vi "LEDTesting.vi"() -> ()   [LabVIEW 2014]
uses:
  <vilib>/myRIO/Instrument Drivers/Onboard IO/DIO/typedefs/DIO Reference.ctl
  <vilib>/myRIO/Common/Instrument Driver Framework/Utilities/typedefs/myRIO Generic Hardware Reference.ctl
  <vilib>/myRIO/Common/Instrument Driver Framework/Utilities/typedefs/Hardware Version Enum.ctl
  <vilib>/myRIO/Common/Instrument Driver Framework/Utilities/typedefs/myRIO v1.0 Reference.ctl
  <vilib>/myRIO/Common/Instrument Driver Framework/Utilities/typedefs/Generic FPGA Reference.ctl
  <vilib>/myRIO/Common/Instrument Driver Framework/myRIO v1.0/DIO/typedefs/DIO Channels List.ctl
  <vilib>/myRIO/Common/Instrument Driver Framework/myRIO v1.0/DIO/typedefs/DIO Channels Enum.ctl
  <vilib>/userdefined/High Color/nirio_resource_hc.ctl
  <vilib>/myRIO/Common/Instrument Driver Framework/Utilities/vis/Is FPGA Ref Available.vi
  <vilib>/myRIO/Common/Instrument Driver Framework/myRIO v1.0/DIO/vis/myRIO v1.1 Open DIO.vi
  <vilib>/myRIO/Instrument Drivers/Onboard IO/DIO/vis/Read.vi
  <vilib>/myRIO/Instrument Drivers/Onboard IO/DIO/vis/Write.vi
  <vilib>/myRIO/Common/Instrument Driver Framework/Utilities/vis/Validate Channels.vi
  <vilib>/myRIO/Common/Instrument Driver Framework/myRIO v1.0/DIO/vis/myRIO v1.0 Reserve DIO.vi
  <vilib>/myRIO/Common/Instrument Driver Framework/myRIO v1.0/Resource Manager/vis/myRIO v1.0 Reserve Channel List.vi
  <vilib>/myRIO/Common/Instrument Driver Framework/myRIO v1.0/DIO/vis/myRIO v1.0 Build MUX Configuration DIO.vi
  <vilib>/myRIO/Common/Instrument Driver Framework/myRIO v1.0/Resource Manager/vis/myRIO v1.0 Reserve Channel.vi
  <vilib>/myRIO/Common/Instrument Driver Framework/myRIO v1.0/Resource Manager/vis/myRIO v1.0 Unreserve Channel.vi
  <vilib>/myRIO/Common/Instrument Driver Framework/myRIO v1.0/Resource Manager/vis/myRIO v1.0 Create Configuration List.vi
  <vilib>/myRIO/Common/Instrument Driver Framework/myRIO v1.0/Resource Manager/vis/myRIO v1.0 Build Mutex Name.vi
  <vilib>/Utility/VariantDataType/GetNumericInfo.vi
  <vilib>/Utility/error.llb/Error Cluster From Error Code.vi
  <vilib>/myRIO/Common/Instrument Driver Framework/myRIO v1.0/myRIO v1.1 Open.vi
  <vilib>/myRIO/Common/Instrument Driver Framework/Utilities/vis/IO Manager.vi
  <vilib>/myRIO/Common/Instrument Driver Framework/Utilities/vis/Configuration Manager.vi
  <vilib>/myRIO/Common/Instrument Driver Framework/myRIO v1.0/Resource Manager/vis/myRIO v1.0 Configure IO.vi
  <vilib>/myRIO/Common/Instrument Driver Framework/myRIO v1.0/myRIO v1.0 Close.vi
  <vilib>/myRIO/Common/Instrument Driver Framework/myRIO v1.0/DIO/vis/myRIO v1.0 Read DIO.vi
  <vilib>/myRIO/Common/Instrument Driver Framework/myRIO v1.0/DIO/vis/myRIO v1.0 Write DIO.vi
  <vilib>/myRIO/Express VI/Onboard IO/DI/DI Express VI.xnode
  <vilib>/myRIO/Instrument Drivers/Onboard IO/DIO/vis/myRIO DIO Open.xnode
  <vilib>/myRIO/Express VI/Onboard IO/DO/DO Express VI.xnode
  <vilib>/myRIO/Instrument Drivers/Onboard IO/DIO/DIO.lvlib
  <vilib>/ptbypt/NI_PtbyPt.lvlib
panel:
  in  "stop":bool
  out "Outlet 1 Mode":enum16{"Off", "On", "Auto"}(ring)=enum."Auto"
  in  "x+1 2":i32
  in  "stop 2":bool
  out "x+1":i32
  in  "Enum":enum16{"Off", "On", "Auto"}(ring)
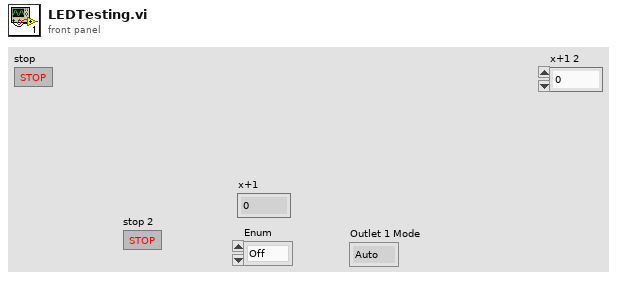
[diagram p1: front panel]
types:
  T1 = typedef "DIO.lvlib/DIO Reference.ctl" = cluster{"myRIO Reference":T2, "DIO Channels List":T6}
  T2 = typedef "myRIO Generic Hardware Reference.ctl" = cluster{"myRIO Model":T3, "myRIO Hardware Reference":T4}
  T3 = typedef "Hardware Version Enum.ctl" = enum16{"Unknown", "myRIO-1900", "myRIO-1950"}
  T4 = typedef "myRIO v1.0 Reference.ctl" = cluster{"Generic FPGA Reference":T5, "Allow multiple opens":bool}
  T5 = typedef "Generic FPGA Reference.ctl" = refnum<k20>
  T6 = typedef "DIO Channels List.ctl" = T7[]
  T7 = typedef "DIO Channels Enum.ctl" = enum16{"Not Connected", "C/DIO0", "C/DIO1", "C/DIO2", "C/DIO3", "C/DIO4", "C/DIO5", "C/DIO6", "C/DIO7", "A/DIO0", "A/DIO1", "A/DIO2", "A/DIO3", "A/DIO4", "A/DIO5", "A/DIO6", "A/DIO7", "A/DIO8", "A/DIO9", "A/DIO10", "A/DIO11", "A/DIO12", "A/DIO13", "A/DIO14", "A/DIO15", "B/DIO0", "B/DIO1", "B/DIO2", "B/DIO3", "B/DIO4", "B/DIO5", "B/DIO6", "B/DIO7", "B/DIO8", "B/DIO9", "B/DIO10", "B/DIO11", "B/DIO12", "B/DIO13", "B/DIO14", "B/DIO15", "LED0", "LED1", "LED2", "LED3", "Button0"}
  T8 = typedef "nirio_resource_hc.ctl" = tag
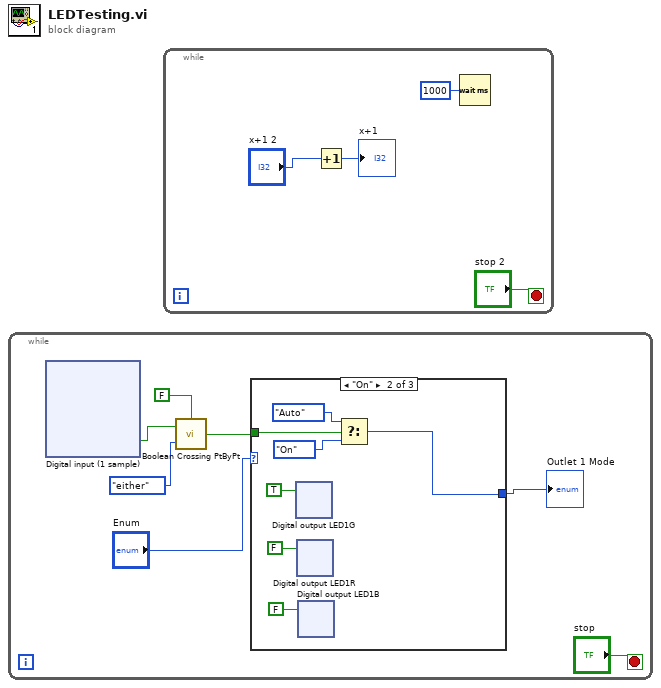
[diagram p0: block diagram]
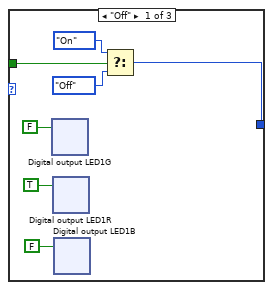
[diagram p2: hidden frame]
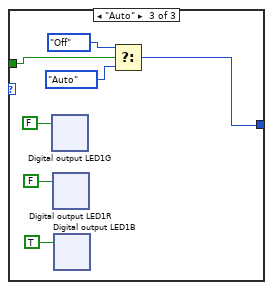
[diagram p3: hidden frame]
diagram:
  n1 = while {
    stop <- "stop" stop-if-true
    n2 = xnode "Digital input (1 sample)"() -> ("Button1 (B/DIO0 (Pin 11))"=w4:bool)  [unwired: 1 in, 1 out]
    n3 = call <vilib>:"Boolean Crossing PtByPt.vi"("initialize"=FALSE, "direction"=enum16{"either", "false-true", "true-false"}."either", "input"=w4) -> ("crossing"=w6:bool)
    n4 = case shown="\"On\"" "Enum" {
      tunnel: [w49 w161 w273] -> w3
      tunnel: w6 -> [w48 w158 w271]
      frame "Off" {
        n5 = xnode "Digital output LED1G"("LED1G (A/DIO0 (Pin 11))"=FALSE) -> ()  [unwired: 1 in, 1 out]
        n6 = xnode "Digital output LED1R"("LED1R (A/DIO1 (Pin 13))"=TRUE) -> ()  [unwired: 1 in, 1 out]
        n7 = xnode "Digital output LED1B"("LED1B (A/DIO2 (Pin 15))"=FALSE) -> ()  [unwired: 1 in, 1 out]
        n8 = Select(t=enum16{"Off", "On", "Auto"}."On", s=w48, f=enum16{"Off", "On", "Auto"}."Off") -> (s? t:f=w49:enum16{"Off", "On", "Auto"})
      }
      frame "On" {
        n9 = xnode "Digital output LED1G"("LED1G (A/DIO0 (Pin 11))"=TRUE) -> ()  [unwired: 1 in, 1 out]
        n10 = xnode "Digital output LED1R"("LED1R (A/DIO1 (Pin 13))"=FALSE) -> ()  [unwired: 1 in, 1 out]
        n11 = xnode "Digital output LED1B"("LED1B (A/DIO2 (Pin 15))"=FALSE) -> ()  [unwired: 1 in, 1 out]
        n12 = Select(t=enum16{"Off", "On", "Auto"}."Auto", s=w158, f=enum16{"Off", "On", "Auto"}."On") -> (s? t:f=w161:enum16{"Off", "On", "Auto"})
      }
      frame "Auto" {
        n13 = xnode "Digital output LED1G"("LED1G (A/DIO0 (Pin 11))"=FALSE) -> ()  [unwired: 1 in, 1 out]
        n14 = xnode "Digital output LED1R"("LED1R (A/DIO1 (Pin 13))"=FALSE) -> ()  [unwired: 1 in, 1 out]
        n15 = xnode "Digital output LED1B"("LED1B (A/DIO2 (Pin 15))"=TRUE) -> ()  [unwired: 1 in, 1 out]
        n16 = Select(t=enum16{"Off", "On", "Auto"}."Off", s=w271, f=enum16{"Off", "On", "Auto"}."Auto") -> (s? t:f=w273:enum16{"Off", "On", "Auto"})
      }
    }
    "Outlet 1 Mode" <- w3
  }
  n17 = while {
    stop <- "stop 2" stop-if-true
    n18 = Increment(x="x+1 2") -> (x+1=→"x+1":i32)
    n19 = Wait (ms)(milliseconds to wait=u32 1000) -> ()  [unwired: 1 out]
  }
